vi "TestExec.Log SW Sync.vi"(8 "error in (no error)":errorcluster, 9 "HistLen":i32=10, 10 "FileName":string="TESyncStatus.txt", 11 "Folder":path) -> (0 "error out":errorcluster)   [LabVIEW 2018]
uses:
  <vilib>/KATE/Files/File Utils.lvlib
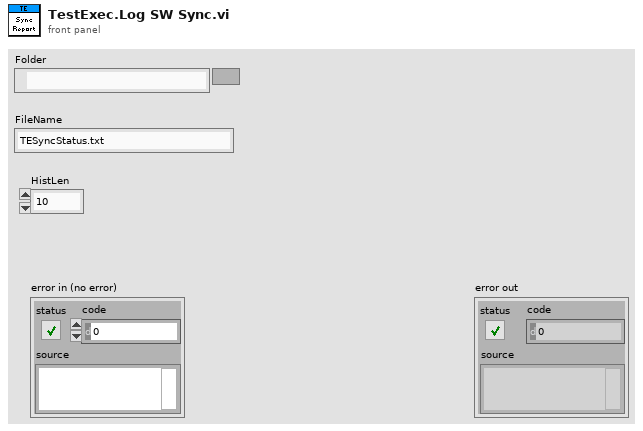
[diagram p1: front panel]
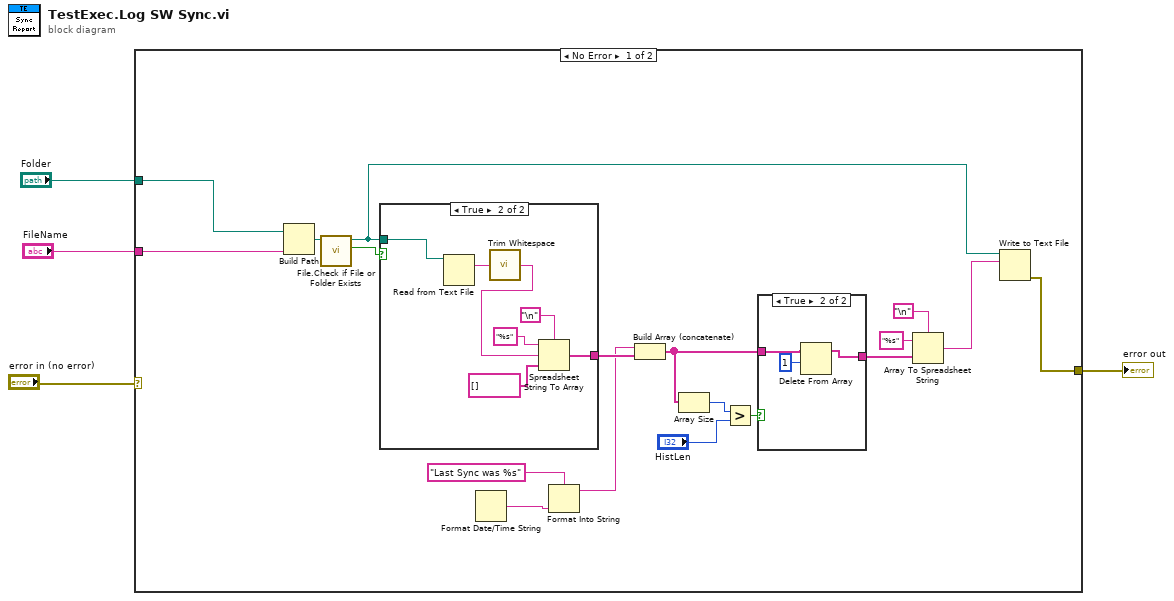
[diagram p0: block diagram]
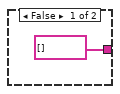
[diagram p2: hidden frame]
diagram:
  n1 = case shown="No Error" "error in (no error)" {
    selector: "error in (no error)" -> [_ w35]
    tunnel: "Folder" -> [w20 _]
    tunnel: "FileName" -> [w19 _]
    tunnel: [w5 w35] -> w2
    frame No Error {
      n2 = Build Path(base path=w20, name or relative path=w19) -> (appended path=w10:path)
      n3 = call <vilib>:"File.Check if File or Folder Exists.vi"("Path"=w10) -> ("Exists"=w9:bool, "Dup Path"=w11:path)  [unwired: 6 in, 3 out]
      n4 = case shown="True" w9 {
        tunnel: [string[] [] ("array type (2D Dbl)") w27] -> w18
        tunnel: w11 -> [_ w26]
        frame False {
        }
        frame True {
          n5 = Read from Text File(file (use dialog)=w26) -> (text=w25:string)  [unwired: 3 in, 3 out]
          n6 = call <vilib>:"Trim Whitespace.vi"("string"=w25) -> ("trimmed string"=w24:string)  [unwired: 1 in]
          n7 = Spreadsheet String To Array(delimiter (Tab)="\n", format string="%s", spreadsheet string=w24, array type (2D Dbl)=string[] []) -> (array=w27:string[])
        }
      }
      n8 = Format Date/Time String() -> (date/time string=w22:string)  [unwired: 3 in]
      n9 = Format Into String(format string="Last Sync was %s", w22) -> (resulting string=w17:string)  [unwired: 2 in, 1 out]
      n10 = Build Array (concatenate)(w17, w18) -> (w16:string[])
      n11 = Array Size(array=w16) -> (size(s)=w8:i32)
      n12 = Greater?(x=w8, y="HistLen") -> (0:w6:bool)
      n13 = case shown="True" w6 {
        tunnel: w16 -> [w31 w34]
        tunnel: [w31 w33] -> w15
        frame False {
        }
        frame True {
          n14 = Delete From Array(array=w34, length=1) -> (array with subset deleted=w33:string[])  [unwired: 1 in, 1 out]
        }
      }
      n15 = Array To Spreadsheet String(delimiter (Tab)="\n", array=w15, 3:"%s" ("format string")) -> (spreadsheet string=w12:string)
      n16 = Write to Text File(file (use dialog)=w11, text=w12) -> (error out=w5:errorcluster)  [unwired: 2 in, 2 out]
    }
    frame Error {
    }
  }
  "error out" <- w2
